vi "获取2号下位机4路温度值并显示.vi"() -> ()   [LabVIEW 2022 SP3]
uses:
  <vilib>/Instr/_visa.llb/VISA Configure Serial Port (Instr).vi
panel:
  out "提取的第四路温度原始数据":string
  out "提取的第三路温度原始数据":string
  out "提取的第二路温度原始数据":string
  out "第一路温度值":dbl[](array[numeric])
  out "提取的第一路温度原始数据":string
  out "获取下位机返回的原始数据包":string
  in  "发送命令":string
  in  "波特率":u32=9600 caption="波特率(9600)"
  in  "选择串口":refnum<visa-resource-name>
  # "第三路温度值"
  # "第四路温度值"
  # "第二路温度值"
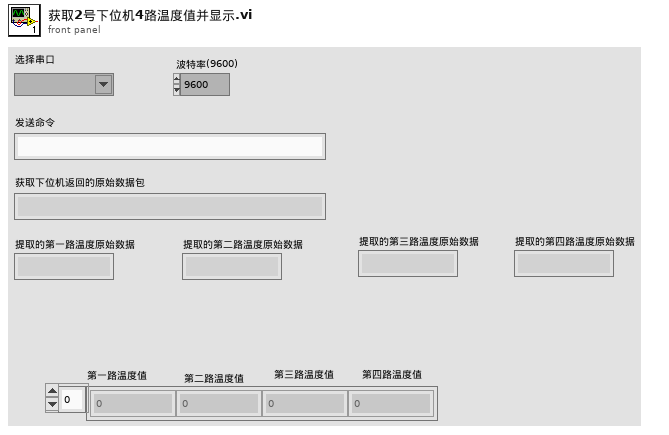
[diagram p1: front panel]
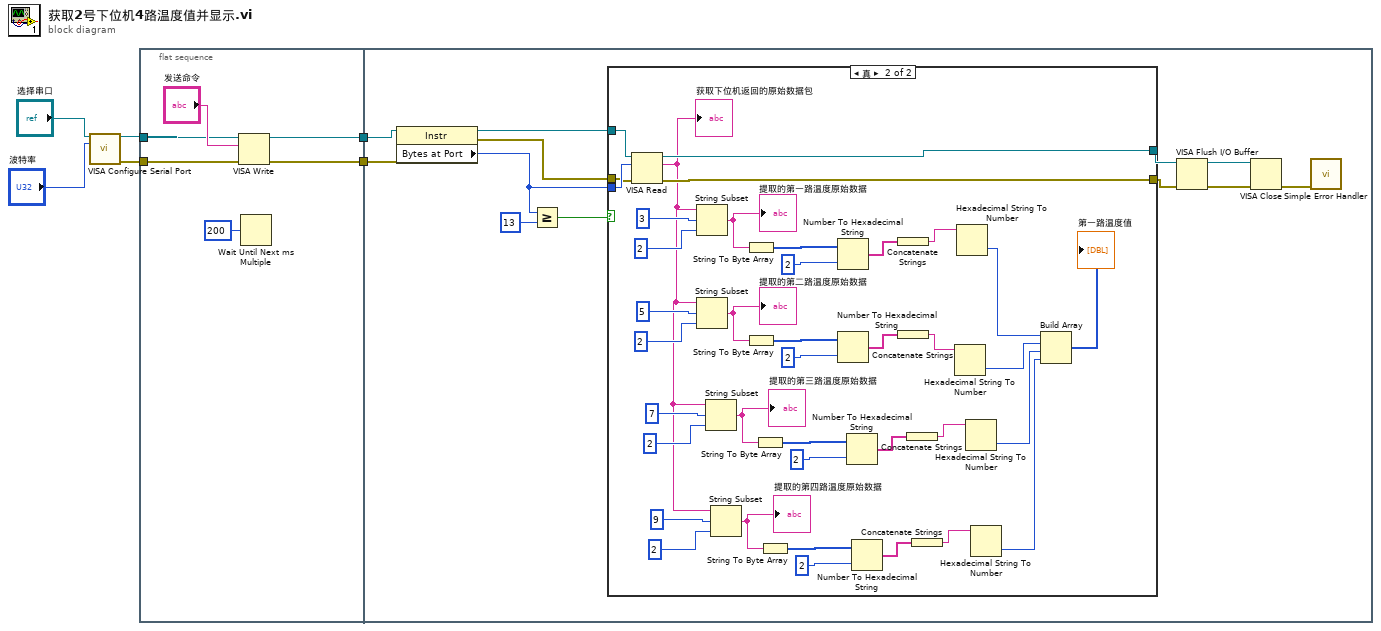
[diagram p0: block diagram]
diagram:
  n1 = call-poly "VISA Configure Serial Port"("VISA resource name"="选择串口", "baud rate (9600)"="波特率") -> ("VISA resource name out"=w4:refnum<visa-resource-name>, "error out"=w3:errorcluster)  [unwired: 12 in]
  n2 = flat-sequence {
    tunnel: w4 -> [w11]
    tunnel: w3 -> [w10]
    tunnel: [w8] -> w2
    tunnel: [w7] -> w1
    tunnel: w2 -> [w24]
    tunnel: w1 -> [w23]
    frame #0 {
      n3 = VISA Write(VISA resource name=w11, write buffer="发送命令", error in (no error)=w10) -> (VISA resource name out=w8:refnum<visa-resource-name>, error out=w7:errorcluster)  [unwired: 1 out]
      n4 = Wait Until Next ms Multiple(millisecond multiple=u32 200 ("毫秒倍数")) -> ()  [unwired: 1 out]
    }
    frame #1 {
      n5 = property class="Instr"(reference=w24, error in=w23) -> (reference out=w20:refnum<visa-resource-name>, error out=w18:errorcluster, "Bytes at Port"=w19:u32)
      n6 = Greater Or Equal?(x=w19, y=u32 13) -> (x >= y?=w22:bool)
      n7 = case shown="真" w22 {
        tunnel: w20 -> [w26 w65]
        tunnel: w19 -> [_ w64]
        tunnel: w18 -> [w25 w63]
        tunnel: [w26 w55] -> w14
        tunnel: [w25 w54] -> w13
        frame False {
        }
        frame True {
          n8 = VISA Read(VISA resource name=w65, byte count=w64, error in (no error)=w63) -> (VISA resource name out=w55:refnum<visa-resource-name>, read buffer=w31:string, error out=w54:errorcluster)  [unwired: 1 out]
          "获取下位机返回的原始数据包" <- w31
          n9 = String Subset(string=w31, offset (0)=3 ("偏移量(0)"), length (rest)=2 ("长度（剩余）")) -> (substring=w60:string)
          "提取的第一路温度原始数据" <- w60
          n10 = String Subset(string=w31, offset (0)=5 ("偏移量(0)"), length (rest)=2 ("长度（剩余）")) -> (substring=w49:string)
          "提取的第二路温度原始数据" <- w49
          n11 = String Subset(string=w31, offset (0)=7 ("偏移量(0)"), length (rest)=2 ("长度（剩余）")) -> (substring=w42:string)
          "提取的第三路温度原始数据" <- w42
          n12 = String Subset(string=w31, offset (0)=9 ("偏移量(0)"), length (rest)=2 ("长度（剩余）")) -> (substring=w36:string)
          "提取的第四路温度原始数据" <- w36
          n13 = String To Byte Array(string=w60) -> (unsigned byte array=w59:u8[])
          n14 = String To Byte Array(string=w49) -> (unsigned byte array=w48:u8[])
          n15 = String To Byte Array(string=w42) -> (unsigned byte array=w41:u8[])
          n16 = String To Byte Array(string=w36) -> (unsigned byte array=w35:u8[])
          n17 = Number To Hexadecimal String(1:i16 2 ("宽度(-)"), 2:w59) -> (0:w57:string[])
          n18 = Number To Hexadecimal String(1:i16 2 ("宽度(-)"), 2:w48) -> (0:w46:string[])
          n19 = Number To Hexadecimal String(1:i16 2 ("宽度(-)"), 2:w41) -> (0:w39:string[])
          n20 = Number To Hexadecimal String(1:i16 2 ("宽度(-)"), 2:w35) -> (0:w33:string[])
          n21 = Concatenate Strings(w57) -> (w56:string)
          n22 = Concatenate Strings(w46) -> (w45:string)
          n23 = Concatenate Strings(w39) -> (w38:string)
          n24 = Concatenate Strings(w33) -> (w32:string)
          n25 = Hexadecimal String To Number(string=w45) -> (number=w29:u32)  [unwired: 2 in, 1 out]
          n26 = Hexadecimal String To Number(string=w56) -> (number=w52:u32)  [unwired: 2 in, 1 out]
          n27 = Hexadecimal String To Number(string=w38) -> (number=w28:u32)  [unwired: 2 in, 1 out]
          n28 = Hexadecimal String To Number(string=w32) -> (number=w27:u32)  [unwired: 2 in, 1 out]
          n29 = Build Array(w52, w29, w28, w27) -> (→"第一路温度值":u32[])
        }
      }
      n30 = VISA Flush I/O Buffer(VISA resource name=w14, error in (no error)=w13) -> (VISA resource name out=w15:refnum<visa-resource-name>, error out=w16:errorcluster)  [unwired: 1 in]
      n31 = VISA Close(VISA resource name=w15, error in (no error)=w16) -> (error out=w17:errorcluster)
      n32 = call <vilib>:"Simple Error Handler.vi"("error in (no error)"=w17) -> ()  [unwired: 4 in, 5 out]
    }
  }
